vi "Show Brief Status.vi"() -> ()   [LabVIEW 2015]
uses:
  Type/_Source Type.ctl
  Type/_RT Command.ctl
  Type/_Log Command.ctl
  Configuration/_Global Configuration.vi
panel:
  out "RT Events":string
  out "HSID Temp:":sgl format="%#.2g"
  out "Exhaust OK":bool
  out "CurGas OK":bool
  out "Pump OK":bool
  out "Interlock OK":bool
  out "Vac. Pressure:":sgl format="%#.2e"
  out "Source 2 Temp:":sgl format="%#.2g"
  out "Source 2 Type:":T1 items=["None", "ESI", "APCI", "APPI", "MicroSpray"]
  out "Source 1 Temp:":sgl format="%#.2g"
  out "Source 1 Type:":T1 items=["None", "ESI", "APCI", "APPI", "MicroSpray"]
  out "Read":bool
  # "Source Status"
  # "Other Status"
  # "Torr"
  # "Interlocks:"
  # "Pump Speed:"
  # "Drying Gas:"
  # "Exhaust Gas:"
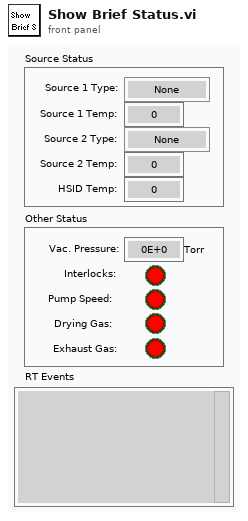
[diagram p1: front panel]
types:
  T1 = typedef "_Source Type.ctl" = i8
  T2 = typedef "_RT Command.ctl" = enum16{"xml Start Run", "xml Start Actual Run", "xml Stop Run", "xml Runtime Update", "xml Get Status", "xml Get Table", "xml Set Table", "xml Get Configuration", "xml System Status", "xml Set LC Input Logic", "xml Get Data", "xml Get Info", "Start", "StartActualRun", "Stop", "Runtime Update", "Get Data", "Get Info", "Get Status", "Get Param", "Get Config", "Get Table", "Read ADC", "Set Oscillator", "Update Config", "Update Table", "Set All Pol", "Set Pol and DC", "Set Max Mass", "Toggle RP", "Toggle EL", "Set PIC", "Initialize Turbo", "Send Turbo Comm", "Close Turbo", "P1", "P2", "P3", "Send Serial", "Set LC Out", "Get LC In", "Read VAC", "Test Table", "Toggle Power", "Get Startup", "Set Startup", "Get ADC Table", "Set ADC Table", "Get Brief Status", "Get Detail Status", "Auxiliary Update", "Set CC Logics", "Set CC Input Logics", "Ignore Error", "invalid"}
  T3 = typedef "_Log Command.ctl" = enum16{"No Command", "Open", "Read", "Write", "Close", "Check Size"}
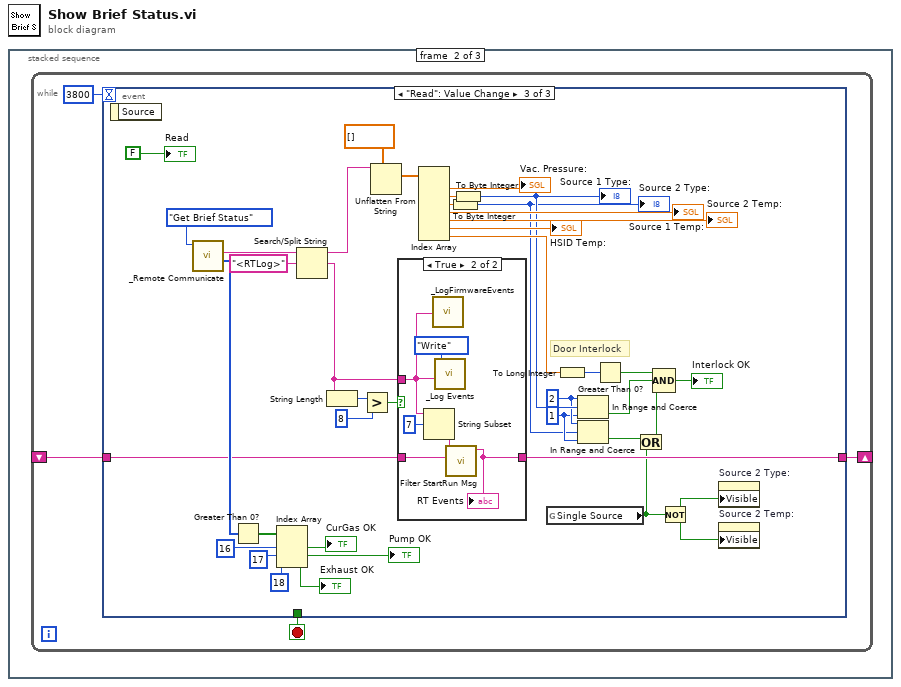
[diagram p0: block diagram]
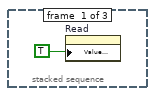
[diagram p2: hidden frame]
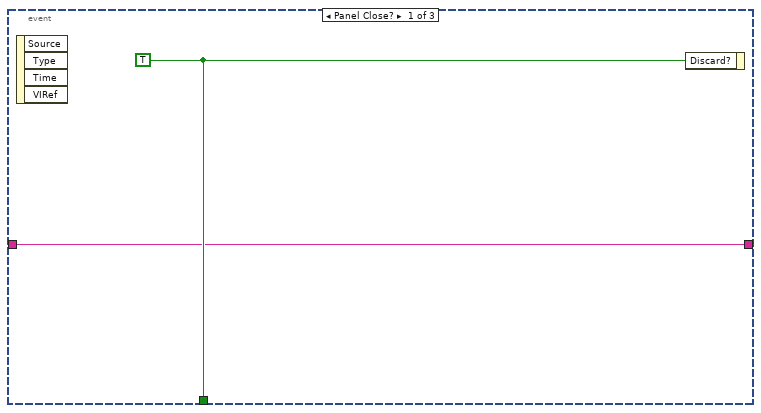
[diagram p3: hidden frame]
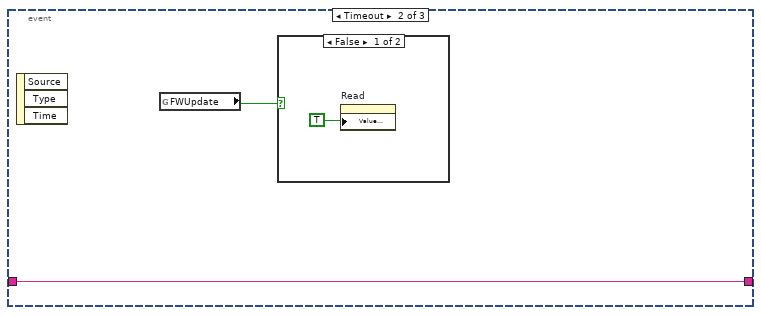
[diagram p4: hidden frame]
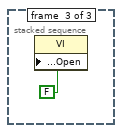
[diagram p7: hidden frame]
diagram:
  n1 = stacked-sequence {
    frame #0 {
      n2 = property on="Read" class="Bool (strict)"("Value (Signaling)"=TRUE) -> ()  [unwired: 2 in, 2 out]
    }
    frame #1 {
      n3 = while {
        shift-right: [w2] -> _
        shift-left: _ -> [w3]
        stop <- w5 stop-if-true
        n4 = event shown="[2] \"Read\": Value Change" {
          selector: _ -> [_ _ _]
          dyn-events: _ -> [_ _ _]
          timeout: 3800 -> [_ _ _]
          tunnel: [w7 _ _] -> w5
          tunnel: w3 -> [w6 w9 w23]
          tunnel: [w6 w9 w22] -> w2
          event Panel Close? {
            w7 = TRUE ("Discard?")
            n5 = event-data() -> ()  [unwired: 5 out]
            n6 = event-data("Discard?"=w7) -> ()  [unwired: 1 in, 1 out]
          }
          event Timeout {
            n7 = event-data() -> ()  [unwired: 4 out]
            n8 = global read "_Global Configuration.vi" "FWUpdate"() -> (w8:bool)
            n9 = case shown="False" w8 {
              frame False {
                n10 = property on="Read" class="Bool (strict)"("Value (Signaling)"=TRUE) -> ()  [unwired: 2 in, 2 out]
              }
              frame True {
              }
            }
          }
          event "Read": Value Change {
            w35 = i8 1 ("lower limit")
            w36 = i8 2 ("upper limit")
            # "Door Interlock"
            n11 = event-data() -> ()  [unwired: 2 out]
            n12 = call "_Remote Communicate.vi"("Command"=_RT_Command."Get Brief Status") -> ("Data Array"=w48:i32[], "Info"=w30:string)  [unwired: 5 in, 2 out]
            n13 = Greater Than 0?(x=w48) -> (x > 0?=w40:bool[])
            n14 = Index Array(array=w40, index #1=16 ("index"), index #2=17 ("index"), index #3=18 ("index")) -> (element #1=→"CurGas OK":bool, element #2=→"Pump OK":bool, element #3=→"Exhaust OK":bool)
            n15 = Search/Split String(string=w30, search string/char (-)="<RTLog>") -> (substring before match=w28:string, match + rest of string=w25:string)  [unwired: 2 out]
            n16 = String Length(string=w25) -> (length=w27:i32)
            n17 = Greater?(x=w27, y=8) -> (0:w24:bool)
            n18 = Unflatten From String(type=sgl[] [], binary string=w28) -> (value=w47:sgl[])  [unwired: 1 in, 4 out]
            n19 = case shown="True" w24 {
              tunnel: w25 -> [_ w55]
              tunnel: w23 -> [w51 w54]
              tunnel: [w51 w53] -> w22
              frame False {
              }
              frame True {
                n20 = String Subset(string=w55, offset (0)=7) -> (substring=w52:string)  [unwired: 1 out]
                n21 = call "_LogFirmwareEvents.vi"("Event"=w55) -> ()
                n22 = call "_Log Events.vi"("Event"=w55, "Log Command"=_Log_Command."Write" ("File Command")) -> ()  [unwired: 6 in, 2 out]
                n23 = call "Filter StartRun Msg.vi"("Current List"=w54, "New RT Events"=w52) -> ("New List"=w53:string)  [unwired: 9 in]
                "RT Events" <- w53
              }
            }
            n24 = Index Array(array=w47) -> (element #1=→"Vac. Pressure:":sgl, element #2=w38:sgl, element #3=w46:sgl, element #4=→"Source 1 Temp:":sgl, element #5=→"Source 2 Temp:":sgl, element #6=→"HSID Temp:":sgl, element #7=w41:sgl)  [unwired: 7 in]
            n25 = To Byte Integer(number=w46) -> (8bit integer=w34:i8)
            "Source 2 Type:" <- w34
            n26 = To Byte Integer(number=w38) -> (8bit integer=w37:i8)
            "Source 1 Type:" <- w37
            n27 = global read "_Global Configuration.vi" "Single Source"() -> (w19:bool)
            n28 = To Long Integer(number=w41) -> (32bit integer=w42:i32)
            n29 = In Range and Coerce(upper limit=w36, x=w37, lower limit=w35) -> (In Range?=w32:bool)  [unwired: 1 out]
            n30 = In Range and Coerce(upper limit=w36, x=w34, lower limit=w35) -> (In Range?=w20:bool)  [unwired: 1 out]
            n31 = Greater Than 0?(x=w42) -> (x > 0?=w33:bool)
            n32 = Or(x=w20, y=w19) -> (x .or. y?=w18:bool)
            n33 = Compound Arithmetic op=AND(w33, w32, w18) -> (→"Interlock OK":bool)
            n34 = Not(x=w19) -> (.not. x?=w21:bool)
            n35 = property on="Source 2 Type:" class="Ring (strict)"("Visible"=w21) -> ()  [unwired: 2 in, 2 out]
            n36 = property on="Source 2 Temp:" class="DigNum (strict)"("Visible"=w21) -> ()  [unwired: 2 in, 2 out]
            "Read" <- FALSE ("Undo")
          }
        }
      }
    }
    frame #2 {
      n37 = property class="VI"("Front Panel.Open"=FALSE ("Front Panel Window:Open")) -> ()  [unwired: 2 in, 2 out]
    }
  }
